vi "Separate Globals from Cal Variables.vi"(0 "Calibration Variables":string[](array[string])) -> (4 "Site Globals":string[](array[string]), 6 "Globals":string[](array[string]))   [LabVIEW 2019]
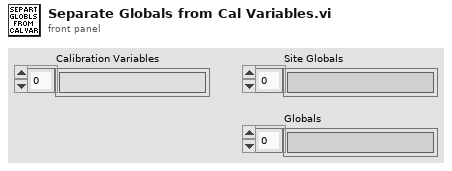
[diagram p1: front panel]
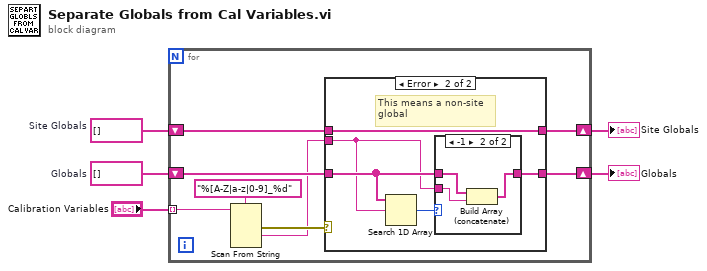
[diagram p0: block diagram]
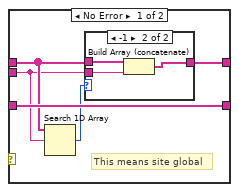
[diagram p2: hidden frame]
diagram:
  w2 = string[] []  # Globals
  w3 = string[] []  # Site Globals
  n1 = for {
    tunnel: "Calibration Variables" -> [w13] mode=indexing
    shift-right: [w8] -> w5
    shift-left: w3 -> [w7]
    shift-right: [w9] -> w1
    shift-left: w2 -> [w10]
    n2 = Scan From String(format string="%[A-Z|a-z|0-9]_%d", input string=w13) -> (error out=w11:errorcluster, output 1=w6:string)  [unwired: 5 in, 2 out]
    n3 = case shown="Error" w11 {
      tunnel: w10 -> [w18 w25]
      tunnel: [w18 w26] -> w9
      tunnel: [w17 w27] -> w8
      tunnel: w7 -> [w15 w27]
      tunnel: w6 -> [w14 w24]
      frame No Error {
        # "This means site global"
        n4 = Search 1D Array(1D array=w15, element=w14) -> (index of element=w16:i32)  [unwired: 1 in]
        n5 = case shown="-1" w16 {
          tunnel: [w19 w22] -> w17
          tunnel: w15 -> [w19 w21]
          tunnel: w14 -> [_ w20]
          frame 0, Default {
          }
          frame -1 {
            n6 = Build Array (concatenate)(w21, w20) -> (w22:string[])
          }
        }
      }
      frame Error {
        # "This means a non-site\nglobal"
        n7 = Search 1D Array(1D array=w25, element=w24) -> (index of element=w23:i32)  [unwired: 1 in]
        n8 = case shown="-1" w23 {
          tunnel: [w28 w31] -> w26
          tunnel: w25 -> [w28 w30]
          tunnel: w24 -> [_ w29]
          frame 0, Default {
          }
          frame -1 {
            n9 = Build Array (concatenate)(w30, w29) -> (w31:string[])
          }
        }
      }
    }
  }
  "Site Globals" <- w5
  "Globals" <- w1
